vi "RT 16 bit ADC DAC.vi"() -> ()   [LabVIEW 2018]
doc: "The myRIO Custom FPGA Project template acquires button data from the onboard button and displays the button value on a Boolean indicator. The SYS.RDY indicator shows the FPGA status."
uses:
  <vilib>/FPGAPlugInAG/myRIO-1900/niLvFpga_Open_myRIO-1900.vi
  <vilib>/rvi/interface/common/dynamic/niFpgaDynamicAddResources.vi
  <vilib>/Utility/error.llb/Error Cluster From Error Code.vi
  <vilib>/rvi/errors/niLvFpgaAdjustHostInterfaceError.vi
  <vilib>/FPGAPlugInAG/Dynamic/niLvFpga_Close_Dynamic.vi
  <vilib>/rvi/interface/nirviOpenFPGA/nirviOpenFPGA.xnode
  PCB Design/16Bit_ADC_DAC/FPGA Bitfiles/ASPE2019StudentC_FPGATarget_FPGASPI_IX3lee3yG5A.lvbitx
  PCB Design/16Bit_ADC_DAC/FPGA_SPI.vi
  <vilib>/rvi/interface/nirviReadWriteControl/nirviReadWriteControl.xnode
  <vilib>/rvi/interface/nirviCloseFPGA/nirviCloseFPGA.xnode
  NiFpgaLv.dll
  <vilib>/rvi/interface/Simulation/niFpgaSimulationCallBeginRW.vi
panel:
  out "avg. loop rate (kHz)":dbl
  in  "time delay":u32=1
  out "G4":dbl(graph)
  out "G3":dbl(graph)
  out "G2":dbl(graph)
  in  "Tab Control":T1(tab)
  in  "CH1":bool[](array[boolean])=[FALSE, FALSE, FALSE, FALSE, FALSE, TRUE, FALSE, FALSE, FALSE, FALSE, FALSE, FALSE, FALSE, FALSE, FALSE, FALSE]
  in  "CH1":bool[](array[boolean])=[FALSE, FALSE, FALSE, TRUE, FALSE, TRUE, FALSE, FALSE, FALSE, FALSE, FALSE, FALSE, FALSE, FALSE, FALSE, FALSE]
  in  "CH2":bool[](array[boolean])=[FALSE, FALSE, FALSE, TRUE, FALSE, TRUE, FALSE, FALSE, FALSE, FALSE, FALSE, FALSE, FALSE, FALSE, FALSE, FALSE]
  in  "CH2":bool[](array[boolean])=[FALSE, FALSE, FALSE, TRUE, FALSE, TRUE, FALSE, FALSE, FALSE, FALSE, FALSE, FALSE, FALSE, FALSE, FALSE, FALSE]
  in  "CH3":bool[](array[boolean])=[FALSE, FALSE, TRUE, FALSE, FALSE, TRUE, FALSE, FALSE, FALSE, FALSE, FALSE, FALSE, FALSE, FALSE, FALSE, FALSE]
  in  "CH1":bool[](array[boolean])=[FALSE, FALSE, FALSE, FALSE, FALSE, TRUE, FALSE, FALSE, FALSE, FALSE, FALSE, FALSE, FALSE, FALSE, FALSE, FALSE]
  in  "CH2":bool[](array[boolean])=[FALSE, FALSE, FALSE, TRUE, FALSE, TRUE, FALSE, FALSE, FALSE, FALSE, FALSE, FALSE, FALSE, FALSE, FALSE, FALSE]
  in  "CH3":bool[](array[boolean])=[FALSE, FALSE, TRUE, FALSE, FALSE, TRUE, FALSE, FALSE, FALSE, FALSE, FALSE, FALSE, FALSE, FALSE, FALSE, FALSE]
  in  "CH4":bool[](array[boolean])=[FALSE, FALSE, TRUE, TRUE, FALSE, TRUE, FALSE, FALSE, FALSE, FALSE, FALSE, FALSE, FALSE, FALSE, FALSE, FALSE]
  in  "CH1":bool[](array[boolean])=[FALSE, FALSE, FALSE, FALSE, FALSE, TRUE, FALSE, FALSE, FALSE, FALSE, FALSE, FALSE, FALSE, FALSE, FALSE, FALSE]
  out "G1":dbl(graph)=0.00030517112470818
  in  "Amplitude":dbl=1.0 format="%0.3p"
  in  "samples per cycle":u32=1000
  out "Freq (kHz)":dbl=0.0007431959564541213 format="%.7g"
  in  "stop":bool
  # "ADC settings:"
  # "DAC settings:"
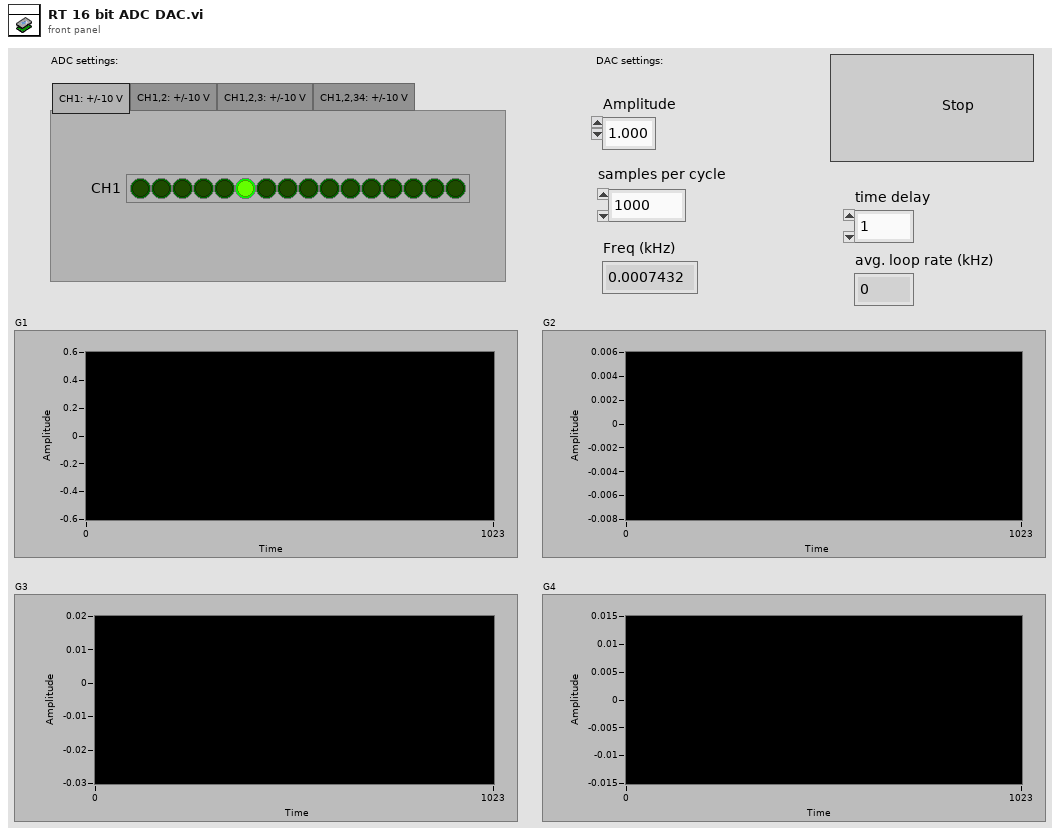
[diagram p1: front panel]
types:
  T1 = enum32{"CH1: +/-10 V", "CH1,2: +/-10 V", "CH1,2,3: +/-10 V", "CH1,2,34: +/-10 V"}
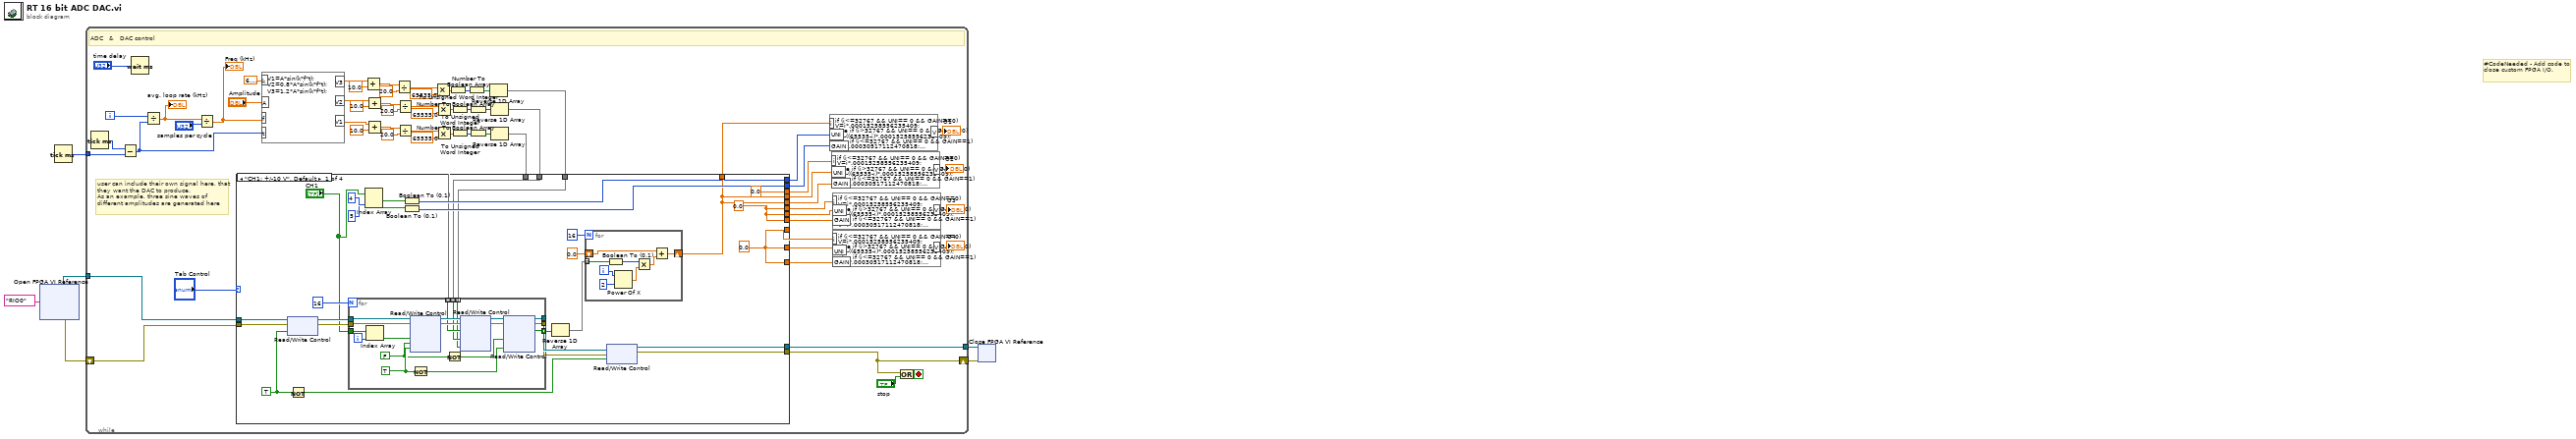
[diagram p0: block diagram]
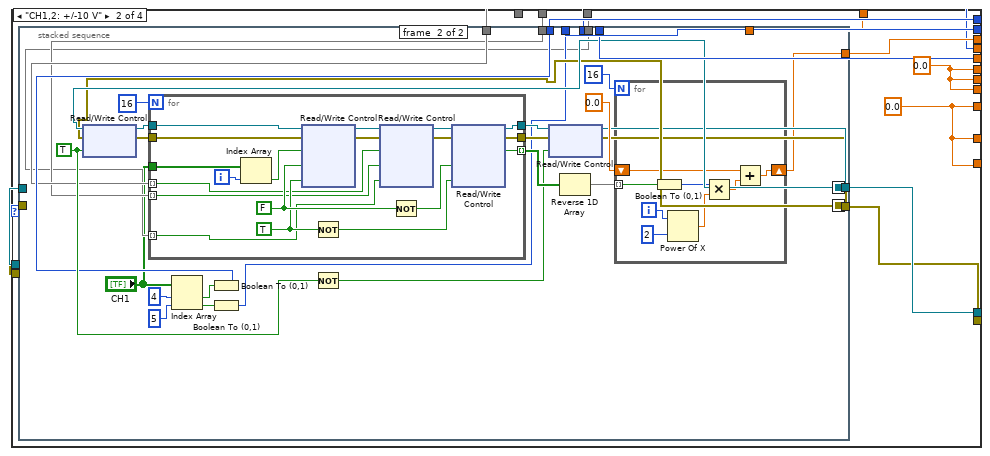
[diagram p2: hidden frame]
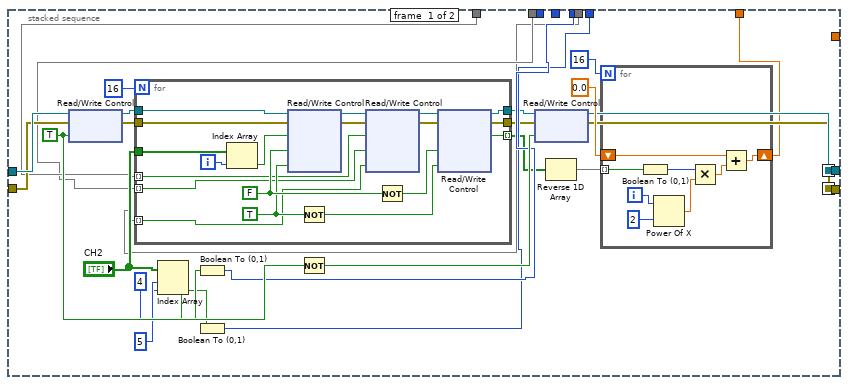
[diagram p3: hidden frame]
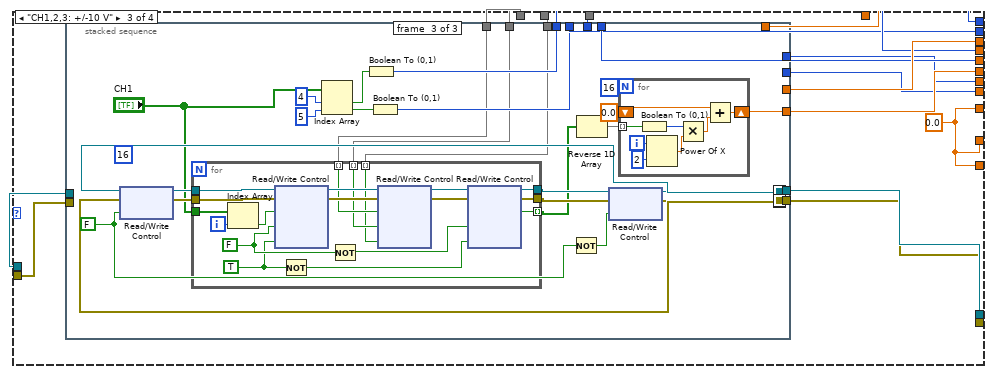
[diagram p4: hidden frame]
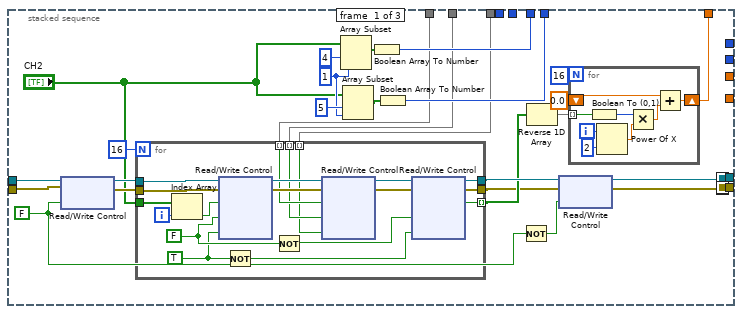
[diagram p5: hidden frame]
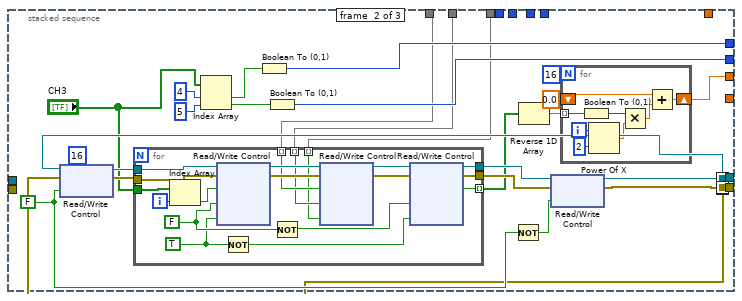
[diagram p6: hidden frame]
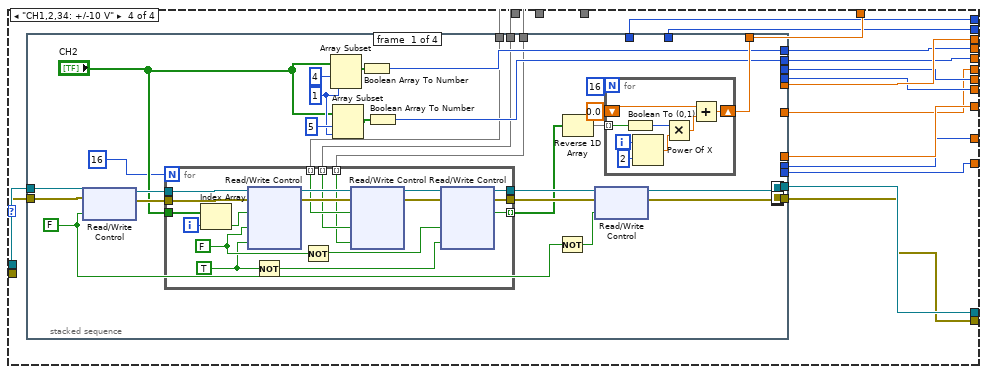
[diagram p7: hidden frame]
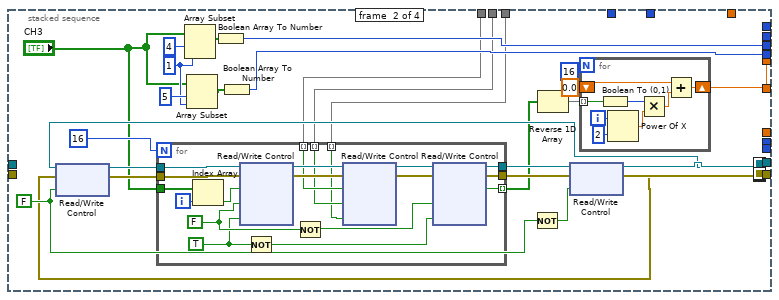
[diagram p8: hidden frame]
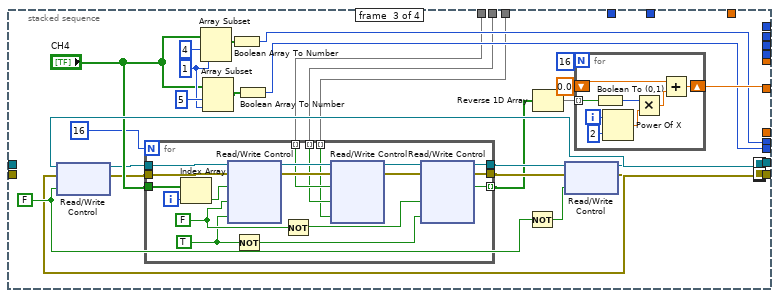
[diagram p9: hidden frame]
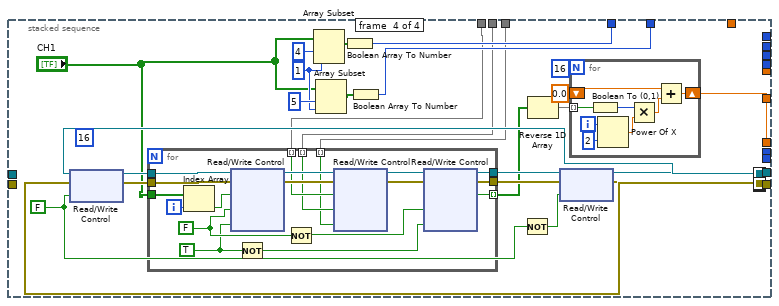
[diagram p10: hidden frame]
diagram:
  # "#CodeNeeded - Add code to close custom FPGA I/O."
  n1 = xnode "Open FPGA VI Reference"("resource name"=tag "RIO0") -> ("FPGA VI Reference Out"=w5:refnum<k20>, "error out"=w4:errorcluster)  [unwired: 1 in]
  n2 = Tick Count (ms)() -> (millisecond timer value=w2:u32)
  n3 = while {
    shift-right: [w56] -> w6
    shift-left: w4 -> [w61]
    tunnel: w2 -> [w67]
    tunnel: w5 -> [w62]
    tunnel: [w57] -> w1
    i -> [w63]
    stop <- w68 stop-if-true
    # "user can include their own signal here, that \nthey want the DAC to produce.\nAs an example, three sine waves of \ndifferent amplitudes are generated here"
    # "ADC   &   DAC control"
    n4 = Tick Count (ms)() -> (millisecond timer value=w65:u32)
    n5 = Subtract(x=w65, y=w67) -> (x-y=w53:u32)
    n6 = Wait (ms)(milliseconds to wait="time delay") -> ()  [unwired: 1 out]
    n7 = Divide(x=w63, y=w53) -> (x/y=w64:dbl)
    "avg. loop rate (kHz)" <- w64
    n8 = Divide(x=w64, y="samples per cycle") -> (x/y=w58:dbl)
    "Freq (kHz)" <- w58
    n9 = formula code="V1=A*sin(k*f*t);\nV2=0.8*A*sin(k*f*t);\nV3=1.2*A*sin(k*f*t);"("t"=w53, "f"=w58, "A"="Amplitude", "k"=6.283185307179586 ("input variable")) -> ("V1"=w25:dbl, "V3"=w44:dbl, "V2"=w34:dbl)
    n10 = Add(x=w44, y=10.0) -> (x+y=w50:dbl)
    n11 = Add(x=w34, y=10.0) -> (x+y=w40:dbl)
    n12 = Add(x=w25, y=10.0) -> (x+y=w31:dbl)
    n13 = Divide(x=w50, y=20.0) -> (x/y=w46:dbl)
    n14 = Divide(x=w40, y=20.0) -> (x/y=w36:dbl)
    n15 = Divide(x=w31, y=20.0) -> (x/y=w27:dbl)
    n16 = Multiply(x=w46, y=65535.0) -> (x*y=w47:dbl)
    n17 = Multiply(x=w36, y=65535.0) -> (x*y=w37:dbl)
    n18 = Multiply(x=w27, y=65535.0) -> (x*y=w28:dbl)
    n19 = To Unsigned Word Integer(number=w47) -> (unsigned 16bit integer=w48:u16)
    n20 = To Unsigned Word Integer(number=w37) -> (unsigned 16bit integer=w38:u16)
    n21 = To Unsigned Word Integer(number=w28) -> (unsigned 16bit integer=w29:u16)
    n22 = Number To Boolean Array(number=w48) -> (Boolean array=w45:bool[])
    n23 = Number To Boolean Array(number=w38) -> (Boolean array=w35:bool[])
    n24 = Number To Boolean Array(number=w29) -> (Boolean array=w26:bool[])
    n25 = Reverse 1D Array(array=w45) -> (reversed array=w43:bool[])
    n26 = Reverse 1D Array(array=w35) -> (reversed array=w24:bool[])
    n27 = Reverse 1D Array(array=w26) -> (reversed array=w23:bool[])
    n28 = case shown="\"CH1: +/-10 V\", Default" "Tab Control" {
      tunnel: w62 -> [w88 w140 w263 w440]
      tunnel: w61 -> [w87 w139 w262 w439]
      tunnel: [w84 w134 w259 w438] -> w22
      tunnel: [w90 w138 w261 w435] -> w57
      tunnel: [w89 w137 w260 w434] -> w56
      tunnel: [0.0 w133 w258 w437] -> w12
      tunnel: [w83 w130 w257 w425] -> w17
      tunnel: [w82 w129 w250 w436] -> w21
      tunnel: [w77 w136 w252 w427] -> w9
      tunnel: [w85 w135 w251 w426] -> w8
      tunnel: [w84 w132 w256 w433] -> w11
      tunnel: [w84 w131 w255 w432] -> w10
      tunnel: [w83 w130 w254 w431] -> w16
      tunnel: [w83 w130 w253 w430] -> w15
      tunnel: [w82 w129 w250 w429] -> w20
      tunnel: [w82 w129 w250 w428] -> w19
      tunnel: w23 -> [w73 w128 w249 w424]
      tunnel: w24 -> [w71 w127 w248 w423]
      tunnel: w43 -> [w70 w126 w247 w422]
      frame "CH1: +/-10 V", Default {
        w82 = 0.0
        w83 = 0.0
        w74 = TRUE ("CS")
        n29 = xnode "Read/Write Control"("FPGA VI Reference In"=w88, "error in"=w87, "CS"=w74) -> ("FPGA VI Reference Out"=w97:refnum<k20>, "error out"=w98:errorcluster)
        n30 = Not(x=w74) -> (.not. x?=w75:bool)
        n31 = for {
          N: 16 -> [_]
          tunnel: w97 -> [w125]
          tunnel: w98 -> [w124]
          tunnel: [w123] -> w96
          tunnel: [w122] -> w95
          tunnel: "CH1" -> [w119]
          tunnel: w73 -> [w112] mode=indexing
          tunnel: [w109] -> w72 mode=indexing
          tunnel: w71 -> [w108] mode=indexing
          tunnel: w70 -> [w107] mode=indexing
          i -> [w121]
          w110 = FALSE ("CLK")
          w114 = TRUE ("CLK")
          n32 = Index Array(array=w119, index=w121) -> (element=w120:bool)
          n33 = xnode "Read/Write Control"("FPGA VI Reference In"=w125, "error in"=w124, "MOSI1"=w120, "CLK2"=w110, "CLK1"=w114) -> ("FPGA VI Reference Out"=w118:refnum<k20>, "error out"=w117:errorcluster)
          n34 = Not(x=w114) -> (.not. x?=w113:bool)
          n35 = Not(x=w110) -> (.not. x?=w111:bool)
          n36 = xnode "Read/Write Control"("FPGA VI Reference In"=w118, "error in"=w117, "MOSI2"=w112, "MOSI3"=w108, "MOSI4"=w107) -> ("FPGA VI Reference Out"=w116:refnum<k20>, "error out"=w115:errorcluster)
          n37 = xnode "Read/Write Control"("FPGA VI Reference In"=w116, "error in"=w115, "CLK2"=w111, "CLK1"=w113) -> ("FPGA VI Reference Out"=w123:refnum<k20>, "error out"=w122:errorcluster, "MISO1"=w109:bool)
        }
        n38 = Index Array(array="CH1", index #1=4 ("index"), index #2=5 ("index")) -> (element #1=w78:bool, element #2=w76:bool)
        n39 = Boolean To (0,1)(Boolean=w78) -> (0, 1=w77:i16)
        n40 = Boolean To (0,1)(Boolean=w76) -> (0, 1=w85:i16)
        n41 = Reverse 1D Array(array=w72) -> (reversed array=w91:bool[])
        n42 = for {
          N: 16 -> [_]
          shift-right: [w104] -> w84
          shift-left: 0.0 -> [w105]
          tunnel: w91 -> [w99] mode=indexing
          i -> [w100]
          n43 = Boolean To (0,1)(Boolean=w99) -> (0, 1=w106:i16)
          n44 = Power Of X(1:2 ("y"), 2:w100) -> (0:w102:dbl)
          n45 = Multiply(x=w106, y=w102) -> (x*y=w103:dbl)
          n46 = Add(x=w105, y=w103) -> (x+y=w104:dbl)
        }
        n47 = xnode "Read/Write Control"("FPGA VI Reference In"=w96, "error in"=w95, "CS"=w75) -> ("FPGA VI Reference Out"=w90:refnum<k20>, "error out"=w89:errorcluster)
      }
      frame "CH1,2: +/-10 V" {
        w129 = 0.0
        w130 = 0.0
        n48 = stacked-sequence {
          seq-local: [w158 _] -> [_ w208]
          seq-local: [w157 _] -> [_ w207]
          tunnel: [w154 _] -> w134
          tunnel: [_ w199] -> w136
          tunnel: [_ w198] -> w135
          tunnel: [_ w204] -> w133
          tunnel: [_ w206] -> w138
          tunnel: [_ w205] -> w137
          tunnel: [w148 _] -> w132
          tunnel: [w147 _] -> w131
          tunnel: w140 -> [w156 _]
          tunnel: w139 -> [w155 _]
          tunnel: w128 -> [w144 w197]
          tunnel: w127 -> [w142 w196]
          tunnel: w126 -> [w141 w195]
          frame #0 {
            w159 = TRUE ("CS")
            n49 = xnode "Read/Write Control"("FPGA VI Reference In"=w156, "error in"=w155, "CS"=w159) -> ("FPGA VI Reference Out"=w165:refnum<k20>, "error out"=w166:errorcluster)
            n50 = for {
              N: 16 -> [_]
              tunnel: w165 -> [w183]
              tunnel: w166 -> [w182]
              tunnel: "CH2" -> [w179]
              tunnel: [w185] -> w146
              tunnel: [w184] -> w145
              tunnel: w144 -> [w181] mode=indexing
              tunnel: [w177] -> w143 mode=indexing
              tunnel: w142 -> [w176] mode=indexing
              tunnel: w141 -> [w175] mode=indexing
              i -> [w180]
              w193 = FALSE ("CLK")
              w192 = TRUE ("CLK")
              n51 = Index Array(array=w179, index=w180) -> (element=w178:bool)
              n52 = xnode "Read/Write Control"("FPGA VI Reference In"=w183, "error in"=w182, "MOSI1"=w178, "CLK2"=w193, "CLK1"=w192) -> ("FPGA VI Reference Out"=w191:refnum<k20>, "error out"=w190:errorcluster)
              n53 = Not(x=w192) -> (.not. x?=w186:bool)
              n54 = xnode "Read/Write Control"("FPGA VI Reference In"=w191, "error in"=w190, "MOSI2"=w181, "MOSI3"=w176, "MOSI4"=w175) -> ("FPGA VI Reference Out"=w189:refnum<k20>, "error out"=w188:errorcluster)
              n55 = Not(x=w193) -> (.not. x?=w187:bool)
              n56 = xnode "Read/Write Control"("FPGA VI Reference In"=w189, "error in"=w188, "CLK2"=w187, "CLK1"=w186) -> ("FPGA VI Reference Out"=w185:refnum<k20>, "error out"=w184:errorcluster, "MISO1"=w177:bool)
            }
            n57 = Index Array(array="CH2", index #1=4 ("index"), index #2=5 ("index")) -> (element #1=w151:bool, element #2=w150:bool)
            n58 = Boolean To (0,1)(Boolean=w151) -> (0, 1=w148:i16)
            n59 = Boolean To (0,1)(Boolean=w150) -> (0, 1=w147:i16)
            n60 = Not(x=w159) -> (.not. x?=w160:bool)
            n61 = xnode "Read/Write Control"("FPGA VI Reference In"=w146, "error in"=w145, "CS"=w160) -> ("FPGA VI Reference Out"=w158:refnum<k20>, "error out"=w157:errorcluster)
            n62 = Reverse 1D Array(array=w143) -> (reversed array=w161:bool[])
            n63 = for {
              N: 16 -> [_]
              shift-right: [w172] -> w154
              shift-left: 0.0 -> [w173]
              tunnel: w161 -> [w167] mode=indexing
              i -> [w168]
              n64 = Boolean To (0,1)(Boolean=w167) -> (0, 1=w174:i16)
              n65 = Power Of X(1:2 ("y"), 2:w168) -> (0:w170:dbl)
              n66 = Multiply(x=w174, y=w170) -> (x*y=w171:dbl)
              n67 = Add(x=w173, y=w171) -> (x+y=w172:dbl)
            }
          }
          frame #1 {
            w209 = TRUE ("CS")
            n68 = xnode "Read/Write Control"("FPGA VI Reference In"=w208, "error in"=w207, "CS"=w209) -> ("FPGA VI Reference Out"=w218:refnum<k20>, "error out"=w219:errorcluster)
            n69 = for {
              N: 16 -> [_]
              tunnel: w218 -> [w246]
              tunnel: w219 -> [w245]
              tunnel: [w244] -> w211 mode=indexing
              tunnel: [w243] -> w217
              tunnel: [w242] -> w216
              tunnel: "CH1" -> [w239]
              tunnel: w197 -> [w232] mode=indexing
              tunnel: w196 -> [w229] mode=indexing
              tunnel: w195 -> [w228] mode=indexing
              i -> [w241]
              w238 = FALSE ("CLK")
              w237 = TRUE ("CLK")
              n70 = Index Array(array=w239, index=w241) -> (element=w240:bool)
              n71 = xnode "Read/Write Control"("FPGA VI Reference In"=w246, "error in"=w245, "MOSI1"=w240, "CLK2"=w238, "CLK1"=w237) -> ("FPGA VI Reference Out"=w236:refnum<k20>, "error out"=w235:errorcluster)
              n72 = Not(x=w237) -> (.not. x?=w230:bool)
              n73 = xnode "Read/Write Control"("FPGA VI Reference In"=w236, "error in"=w235, "MOSI2"=w232, "MOSI3"=w229, "MOSI4"=w228) -> ("FPGA VI Reference Out"=w234:refnum<k20>, "error out"=w233:errorcluster)
              n74 = Not(x=w238) -> (.not. x?=w231:bool)
              n75 = xnode "Read/Write Control"("FPGA VI Reference In"=w234, "error in"=w233, "CLK2"=w231, "CLK1"=w230) -> ("FPGA VI Reference Out"=w243:refnum<k20>, "error out"=w242:errorcluster, "MISO1"=w244:bool)
            }
            n76 = Index Array(array="CH1", index #1=4 ("index"), index #2=5 ("index")) -> (element #1=w201:bool, element #2=w200:bool)
            n77 = Boolean To (0,1)(Boolean=w201) -> (0, 1=w199:i16)
            n78 = Boolean To (0,1)(Boolean=w200) -> (0, 1=w198:i16)
            n79 = Not(x=w209) -> (.not. x?=w210:bool)
            n80 = xnode "Read/Write Control"("FPGA VI Reference In"=w217, "error in"=w216, "CS"=w210) -> ("FPGA VI Reference Out"=w206:refnum<k20>, "error out"=w205:errorcluster)
            n81 = Reverse 1D Array(array=w211) -> (reversed array=w212:bool[])
            n82 = for {
              N: 16 -> [_]
              shift-right: [w225] -> w204
              shift-left: 0.0 -> [w226]
              tunnel: w212 -> [w220] mode=indexing
              i -> [w221]
              n83 = Boolean To (0,1)(Boolean=w220) -> (0, 1=w227:i16)
              n84 = Power Of X(1:2 ("y"), 2:w221) -> (0:w223:dbl)
              n85 = Multiply(x=w227, y=w223) -> (x*y=w224:dbl)
              n86 = Add(x=w226, y=w224) -> (x+y=w225:dbl)
            }
          }
        }
      }
      frame "CH1,2,3: +/-10 V" {
        w250 = 0.0
        n87 = stacked-sequence {
          seq-local: [w285 _ _] -> [_ w335 _]
          seq-local: [w284 _ _] -> [_ w334 _]
          seq-local: [_ w337 _] -> [_ _ w389]
          seq-local: [_ w336 _] -> [_ _ w388]
          tunnel: [w283 _ _] -> w259
          tunnel: [_ w333 _] -> w258
          tunnel: [_ _ w387] -> w261
          tunnel: [_ _ w386] -> w260
          tunnel: [_ _ w385] -> w257
          tunnel: w263 -> [w282 _ _]
          tunnel: w262 -> [w281 _ _]
          tunnel: [w275 _ _] -> w256
          tunnel: [w274 _ _] -> w255
          tunnel: [_ w328 _] -> w254
          tunnel: [_ w327 _] -> w253
          tunnel: [_ _ w384] -> w252
          tunnel: [_ _ w383] -> w251
          tunnel: w249 -> [w270 w320 w375]
          tunnel: w248 -> [w265 w319 w371]
          tunnel: w247 -> [w264 w318 w370]
          frame #0 {
            w276 = 1 ("length")
            w286 = FALSE ("CS")
            n88 = xnode "Read/Write Control"("FPGA VI Reference In"=w282, "error in"=w281, "CS"=w286) -> ("FPGA VI Reference Out"=w273:refnum<k20>, "error out"=w272:errorcluster)
            n89 = for {
              N: 16 -> [_]
              tunnel: w273 -> [w309]
              tunnel: w272 -> [w308]
              tunnel: [w307] -> w268 mode=indexing
              tunnel: [w306] -> w269
              tunnel: [w305] -> w267
              tunnel: "CH2" -> [w302]
              tunnel: w270 -> [w295] mode=indexing
              tunnel: w265 -> [w292] mode=indexing
              tunnel: w264 -> [w291] mode=indexing
              i -> [w304]
              w301 = FALSE ("CLK")
              w300 = TRUE ("CLK")
              n90 = Index Array(array=w302, index=w304) -> (element=w303:bool)
              n91 = xnode "Read/Write Control"("FPGA VI Reference In"=w309, "error in"=w308, "MOSI1"=w303, "CLK2"=w301, "CLK1"=w300) -> ("FPGA VI Reference Out"=w299:refnum<k20>, "error out"=w298:errorcluster)
              n92 = Not(x=w300) -> (.not. x?=w293:bool)
              n93 = Not(x=w301) -> (.not. x?=w294:bool)
              n94 = xnode "Read/Write Control"("FPGA VI Reference In"=w299, "error in"=w298, "MOSI2"=w295, "MOSI3"=w292, "MOSI4"=w291) -> ("FPGA VI Reference Out"=w297:refnum<k20>, "error out"=w296:errorcluster)
              n95 = xnode "Read/Write Control"("FPGA VI Reference In"=w297, "error in"=w296, "CLK2"=w294, "CLK1"=w293) -> ("FPGA VI Reference Out"=w306:refnum<k20>, "error out"=w305:errorcluster, "MISO1"=w307:bool)
            }
            n96 = Array Subset(array="CH2", index=4, length=w276) -> (w278:bool[])
            n97 = Array Subset(array="CH2", index=5, length=w276) -> (w277:bool[])
            n98 = Boolean Array To Number(Boolean array=w278) -> (number=w275:u32)
            n99 = Boolean Array To Number(Boolean array=w277) -> (number=w274:u32)
            n100 = Not(x=w286) -> (.not. x?=w287:bool)
            n101 = Reverse 1D Array(array=w268) -> (reversed array=w288:bool[])
            n102 = xnode "Read/Write Control"("FPGA VI Reference In"=w269, "error in"=w267, "CS"=w287) -> ("FPGA VI Reference Out"=w285:refnum<k20>, "error out"=w284:errorcluster)
            n103 = for {
              N: 16 -> [_]
              shift-right: [w310] -> w283
              shift-left: 0.0 -> [w316]
              tunnel: w288 -> [w311] mode=indexing
              i -> [w312]
              n104 = Boolean To (0,1)(Boolean=w311) -> (0, 1=w317:i16)
              n105 = Power Of X(1:2 ("y"), 2:w312) -> (0:w314:dbl)
              n106 = Multiply(x=w317, y=w314) -> (x*y=w315:dbl)
              n107 = Add(x=w316, y=w315) -> (x+y=w310:dbl)
            }
          }
          frame #1 {
            w338 = FALSE ("CS")
            (unwired) 16
            n108 = xnode "Read/Write Control"("FPGA VI Reference In"=w335, "error in"=w334, "CS"=w338) -> ("FPGA VI Reference Out"=w326:refnum<k20>, "error out"=w325:errorcluster)
            n109 = for {
              tunnel: w326 -> [w361]
              tunnel: w325 -> [w360]
              tunnel: [w359] -> w321 mode=indexing
              tunnel: [w358] -> w323
              tunnel: [w357] -> w322
              tunnel: "CH3" -> [w354]
              tunnel: w320 -> [w347] mode=indexing
              tunnel: w319 -> [w344] mode=indexing
              tunnel: w318 -> [w343] mode=indexing
              i -> [w356]
              w353 = FALSE ("CLK")
              w352 = TRUE ("CLK")
              n110 = Index Array(array=w354, index=w356) -> (element=w355:bool)
              n111 = xnode "Read/Write Control"("FPGA VI Reference In"=w361, "error in"=w360, "MOSI1"=w355, "CLK2"=w353, "CLK1"=w352) -> ("FPGA VI Reference Out"=w351:refnum<k20>, "error out"=w350:errorcluster)
              n112 = Not(x=w352) -> (.not. x?=w345:bool)
              n113 = Not(x=w353) -> (.not. x?=w346:bool)
              n114 = xnode "Read/Write Control"("FPGA VI Reference In"=w351, "error in"=w350, "MOSI2"=w347, "MOSI3"=w344, "MOSI4"=w343) -> ("FPGA VI Reference Out"=w349:refnum<k20>, "error out"=w348:errorcluster)
              n115 = xnode "Read/Write Control"("FPGA VI Reference In"=w349, "error in"=w348, "CLK2"=w346, "CLK1"=w345) -> ("FPGA VI Reference Out"=w358:refnum<k20>, "error out"=w357:errorcluster, "MISO1"=w359:bool)
            }
            n116 = Index Array(array="CH3", index #1=4 ("index"), index #2=5 ("index")) -> (element #1=w330:bool, element #2=w329:bool)
            n117 = Boolean To (0,1)(Boolean=w330) -> (0, 1=w328:i16)
            n118 = Boolean To (0,1)(Boolean=w329) -> (0, 1=w327:i16)
            n119 = Not(x=w338) -> (.not. x?=w339:bool)
            n120 = Reverse 1D Array(array=w321) -> (reversed array=w340:bool[])
            n121 = xnode "Read/Write Control"("FPGA VI Reference In"=w323, "error in"=w322, "CS"=w339) -> ("FPGA VI Reference Out"=w337:refnum<k20>, "error out"=w336:errorcluster)
            n122 = for {
              N: 16 -> [_]
              shift-right: [w367] -> w333
              shift-left: 0.0 -> [w368]
              tunnel: w340 -> [w362] mode=indexing
              i -> [w363]
              n123 = Boolean To (0,1)(Boolean=w362) -> (0, 1=w369:i16)
              n124 = Power Of X(1:2 ("y"), 2:w363) -> (0:w365:dbl)
              n125 = Multiply(x=w369, y=w365) -> (x*y=w366:dbl)
              n126 = Add(x=w368, y=w366) -> (x+y=w367:dbl)
            }
          }
          frame #2 {
            w390 = FALSE ("CS")
            (unwired) 16
            n127 = xnode "Read/Write Control"("FPGA VI Reference In"=w389, "error in"=w388, "CS"=w390) -> ("FPGA VI Reference Out"=w374:refnum<k20>, "error out"=w373:errorcluster)
            n128 = for {
              tunnel: w374 -> [w413]
              tunnel: w373 -> [w412]
              tunnel: [w411] -> w376 mode=indexing
              tunnel: [w410] -> w378
              tunnel: [w409] -> w377
              tunnel: "CH1" -> [w406]
              tunnel: w375 -> [w399] mode=indexing
              tunnel: w371 -> [w396] mode=indexing
              tunnel: w370 -> [w395] mode=indexing
              i -> [w408]
              w405 = FALSE ("CLK")
              w404 = TRUE ("CLK")
              n129 = Index Array(array=w406, index=w408) -> (element=w407:bool)
              n130 = xnode "Read/Write Control"("FPGA VI Reference In"=w413, "error in"=w412, "MOSI1"=w407, "CLK2"=w405, "CLK1"=w404) -> ("FPGA VI Reference Out"=w403:refnum<k20>, "error out"=w402:errorcluster)
              n131 = Not(x=w404) -> (.not. x?=w397:bool)
              n132 = Not(x=w405) -> (.not. x?=w398:bool)
              n133 = xnode "Read/Write Control"("FPGA VI Reference In"=w403, "error in"=w402, "MOSI2"=w399, "MOSI3"=w396, "MOSI4"=w395) -> ("FPGA VI Reference Out"=w401:refnum<k20>, "error out"=w400:errorcluster)
              n134 = xnode "Read/Write Control"("FPGA VI Reference In"=w401, "error in"=w400, "CLK2"=w398, "CLK1"=w397) -> ("FPGA VI Reference Out"=w410:refnum<k20>, "error out"=w409:errorcluster, "MISO1"=w411:bool)
            }
            n135 = Index Array(array="CH1", index #1=4 ("index"), index #2=5 ("index")) -> (element #1=w380:bool, element #2=w379:bool)
            n136 = Boolean To (0,1)(Boolean=w380) -> (0, 1=w384:i16)
            n137 = Boolean To (0,1)(Boolean=w379) -> (0, 1=w383:i16)
            n138 = Not(x=w390) -> (.not. x?=w391:bool)
            n139 = Reverse 1D Array(array=w376) -> (reversed array=w392:bool[])
            n140 = xnode "Read/Write Control"("FPGA VI Reference In"=w378, "error in"=w377, "CS"=w391) -> ("FPGA VI Reference Out"=w387:refnum<k20>, "error out"=w386:errorcluster)
            n141 = for {
              N: 16 -> [_]
              shift-right: [w419] -> w385
              shift-left: 0.0 -> [w420]
              tunnel: w392 -> [w414] mode=indexing
              i -> [w415]
              n142 = Boolean To (0,1)(Boolean=w414) -> (0, 1=w421:i16)
              n143 = Power Of X(1:2 ("y"), 2:w415) -> (0:w417:dbl)
              n144 = Multiply(x=w421, y=w417) -> (x*y=w418:dbl)
              n145 = Add(x=w420, y=w418) -> (x+y=w419:dbl)
            }
          }
        }
      }
      frame "CH1,2,34: +/-10 V" {
        n146 = stacked-sequence {
          seq-local: [w462 _ _ _] -> [_ w514 _ _]
          seq-local: [w461 _ _ _] -> [_ w513 _ _]
          seq-local: [_ w516 _ _] -> [_ _ w570 _]
          seq-local: [_ w515 _ _] -> [_ _ w569 _]
          seq-local: [_ _ w568 _] -> [_ _ _ w623]
          seq-local: [_ _ w567 _] -> [_ _ _ w622]
          tunnel: [w460 _ _ _] -> w438
          tunnel: [_ w512 _ _] -> w437
          tunnel: [_ _ w566 _] -> w425
          tunnel: [_ _ _ w621] -> w435
          tunnel: [_ _ _ w620] -> w434
          tunnel: [_ _ _ w619] -> w436
          tunnel: w440 -> [w459 _ _ _]
          tunnel: w439 -> [w458 _ _ _]
          tunnel: [w452 _ _ _] -> w433
          tunnel: [w451 _ _ _] -> w432
          tunnel: [_ w506 _ _] -> w431
          tunnel: [_ w505 _ _] -> w430
          tunnel: [_ _ w560 _] -> w429
          tunnel: [_ _ w559 _] -> w428
          tunnel: [_ _ _ w613] -> w427
          tunnel: [_ _ _ w612] -> w426
          tunnel: w424 -> [w446 w500 w554 w608]
          tunnel: w423 -> [w442 w496 w550 w604]
          tunnel: w422 -> [w441 w495 w549 w603]
          frame #0 {
            w453 = 1 ("length")
            w463 = FALSE ("CS")
            n147 = xnode "Read/Write Control"("FPGA VI Reference In"=w459, "error in"=w458, "CS"=w463) -> ("FPGA VI Reference Out"=w450:refnum<k20>, "error out"=w449:errorcluster)
            n148 = for {
              N: 16 -> [_]
              tunnel: w450 -> [w486]
              tunnel: w449 -> [w485]
              tunnel: [w484] -> w443 mode=indexing
              tunnel: [w483] -> w445
              tunnel: [w482] -> w444
              tunnel: "CH2" -> [w479]
              tunnel: w446 -> [w472] mode=indexing
              tunnel: w442 -> [w469] mode=indexing
              tunnel: w441 -> [w468] mode=indexing
              i -> [w481]
              w478 = FALSE ("CLK")
              w477 = TRUE ("CLK")
              n149 = Index Array(array=w479, index=w481) -> (element=w480:bool)
              n150 = xnode "Read/Write Control"("FPGA VI Reference In"=w486, "error in"=w485, "MOSI1"=w480, "CLK2"=w478, "CLK1"=w477) -> ("FPGA VI Reference Out"=w476:refnum<k20>, "error out"=w475:errorcluster)
              n151 = Not(x=w477) -> (.not. x?=w470:bool)
              n152 = Not(x=w478) -> (.not. x?=w471:bool)
              n153 = xnode "Read/Write Control"("FPGA VI Reference In"=w476, "error in"=w475, "MOSI2"=w472, "MOSI3"=w469, "MOSI4"=w468) -> ("FPGA VI Reference Out"=w474:refnum<k20>, "error out"=w473:errorcluster)
              n154 = xnode "Read/Write Control"("FPGA VI Reference In"=w474, "error in"=w473, "CLK2"=w471, "CLK1"=w470) -> ("FPGA VI Reference Out"=w483:refnum<k20>, "error out"=w482:errorcluster, "MISO1"=w484:bool)
            }
            n155 = Array Subset(array="CH2", index=4, length=w453) -> (w455:bool[])
            n156 = Array Subset(array="CH2", index=5, length=w453) -> (w454:bool[])
            n157 = Boolean Array To Number(Boolean array=w455) -> (number=w452:u32)
            n158 = Boolean Array To Number(Boolean array=w454) -> (number=w451:u32)
            n159 = Not(x=w463) -> (.not. x?=w464:bool)
            n160 = Reverse 1D Array(array=w443) -> (reversed array=w465:bool[])
            n161 = xnode "Read/Write Control"("FPGA VI Reference In"=w445, "error in"=w444, "CS"=w464) -> ("FPGA VI Reference Out"=w462:refnum<k20>, "error out"=w461:errorcluster)
            n162 = for {
              N: 16 -> [_]
              shift-right: [w492] -> w460
              shift-left: 0.0 -> [w493]
              tunnel: w465 -> [w487] mode=indexing
              i -> [w488]
              n163 = Boolean To (0,1)(Boolean=w487) -> (0, 1=w494:i16)
              n164 = Power Of X(1:2 ("y"), 2:w488) -> (0:w490:dbl)
              n165 = Multiply(x=w494, y=w490) -> (x*y=w491:dbl)
              n166 = Add(x=w493, y=w491) -> (x+y=w492:dbl)
            }
          }
          frame #1 {
            w507 = 1 ("length")
            w517 = FALSE ("CS")
            n167 = xnode "Read/Write Control"("FPGA VI Reference In"=w514, "error in"=w513, "CS"=w517) -> ("FPGA VI Reference Out"=w499:refnum<k20>, "error out"=w498:errorcluster)
            n168 = for {
              N: 16 -> [_]
              tunnel: w499 -> [w540]
              tunnel: w498 -> [w539]
              tunnel: [w538] -> w501 mode=indexing
              tunnel: [w537] -> w503
              tunnel: [w536] -> w502
              tunnel: "CH3" -> [w533]
              tunnel: w500 -> [w526] mode=indexing
              tunnel: w496 -> [w523] mode=indexing
              tunnel: w495 -> [w522] mode=indexing
              i -> [w535]
              w532 = FALSE ("CLK")
              w531 = TRUE ("CLK")
              n169 = Index Array(array=w533, index=w535) -> (element=w534:bool)
              n170 = xnode "Read/Write Control"("FPGA VI Reference In"=w540, "error in"=w539, "MOSI1"=w534, "CLK2"=w532, "CLK1"=w531) -> ("FPGA VI Reference Out"=w530:refnum<k20>, "error out"=w529:errorcluster)
              n171 = Not(x=w531) -> (.not. x?=w524:bool)
              n172 = Not(x=w532) -> (.not. x?=w525:bool)
              n173 = xnode "Read/Write Control"("FPGA VI Reference In"=w530, "error in"=w529, "MOSI2"=w526, "MOSI3"=w523, "MOSI4"=w522) -> ("FPGA VI Reference Out"=w528:refnum<k20>, "error out"=w527:errorcluster)
              n174 = xnode "Read/Write Control"("FPGA VI Reference In"=w528, "error in"=w527, "CLK2"=w525, "CLK1"=w524) -> ("FPGA VI Reference Out"=w537:refnum<k20>, "error out"=w536:errorcluster, "MISO1"=w538:bool)
            }
            n175 = Array Subset(array="CH3", index=4, length=w507) -> (w509:bool[])
            n176 = Array Subset(array="CH3", index=5, length=w507) -> (w508:bool[])
            n177 = Boolean Array To Number(Boolean array=w509) -> (number=w506:u32)
            n178 = Boolean Array To Number(Boolean array=w508) -> (number=w505:u32)
            n179 = Not(x=w517) -> (.not. x?=w518:bool)
            n180 = Reverse 1D Array(array=w501) -> (reversed array=w519:bool[])
            n181 = xnode "Read/Write Control"("FPGA VI Reference In"=w503, "error in"=w502, "CS"=w518) -> ("FPGA VI Reference Out"=w516:refnum<k20>, "error out"=w515:errorcluster)
            n182 = for {
              N: 16 -> [_]
              shift-right: [w546] -> w512
              shift-left: 0.0 -> [w547]
              tunnel: w519 -> [w541] mode=indexing
              i -> [w542]
              n183 = Boolean To (0,1)(Boolean=w541) -> (0, 1=w548:i16)
              n184 = Power Of X(1:2 ("y"), 2:w542) -> (0:w544:dbl)
              n185 = Multiply(x=w548, y=w544) -> (x*y=w545:dbl)
              n186 = Add(x=w547, y=w545) -> (x+y=w546:dbl)
            }
          }
          frame #2 {
            w561 = 1 ("length")
            w571 = FALSE ("CS")
            n187 = xnode "Read/Write Control"("FPGA VI Reference In"=w570, "error in"=w569, "CS"=w571) -> ("FPGA VI Reference Out"=w556:refnum<k20>, "error out"=w557:errorcluster)
            n188 = for {
              N: 16 -> [_]
              tunnel: w556 -> [w594]
              tunnel: w557 -> [w593]
              tunnel: [w592] -> w551 mode=indexing
              tunnel: [w591] -> w553
              tunnel: [w590] -> w552
              tunnel: "CH4" -> [w587]
              tunnel: w554 -> [w580] mode=indexing
              tunnel: w550 -> [w577] mode=indexing
              tunnel: w549 -> [w576] mode=indexing
              i -> [w589]
              w586 = FALSE ("CLK")
              w585 = TRUE ("CLK")
              n189 = Index Array(array=w587, index=w589) -> (element=w588:bool)
              n190 = xnode "Read/Write Control"("FPGA VI Reference In"=w594, "error in"=w593, "MOSI1"=w588, "CLK2"=w586, "CLK1"=w585) -> ("FPGA VI Reference Out"=w584:refnum<k20>, "error out"=w583:errorcluster)
              n191 = Not(x=w585) -> (.not. x?=w578:bool)
              n192 = Not(x=w586) -> (.not. x?=w579:bool)
              n193 = xnode "Read/Write Control"("FPGA VI Reference In"=w584, "error in"=w583, "MOSI2"=w580, "MOSI3"=w577, "MOSI4"=w576) -> ("FPGA VI Reference Out"=w582:refnum<k20>, "error out"=w581:errorcluster)
              n194 = xnode "Read/Write Control"("FPGA VI Reference In"=w582, "error in"=w581, "CLK2"=w579, "CLK1"=w578) -> ("FPGA VI Reference Out"=w591:refnum<k20>, "error out"=w590:errorcluster, "MISO1"=w592:bool)
            }
            n195 = Array Subset(array="CH4", index=4, length=w561) -> (w563:bool[])
            n196 = Array Subset(array="CH4", index=5, length=w561) -> (w562:bool[])
            n197 = Boolean Array To Number(Boolean array=w563) -> (number=w560:u32)
            n198 = Boolean Array To Number(Boolean array=w562) -> (number=w559:u32)
            n199 = Not(x=w571) -> (.not. x?=w572:bool)
            n200 = Reverse 1D Array(array=w551) -> (reversed array=w573:bool[])
            n201 = xnode "Read/Write Control"("FPGA VI Reference In"=w553, "error in"=w552, "CS"=w572) -> ("FPGA VI Reference Out"=w568:refnum<k20>, "error out"=w567:errorcluster)
            n202 = for {
              N: 16 -> [_]
              shift-right: [w600] -> w566
              shift-left: 0.0 -> [w601]
              tunnel: w573 -> [w595] mode=indexing
              i -> [w596]
              n203 = Boolean To (0,1)(Boolean=w595) -> (0, 1=w602:i16)
              n204 = Power Of X(1:2 ("y"), 2:w596) -> (0:w598:dbl)
              n205 = Multiply(x=w602, y=w598) -> (x*y=w599:dbl)
              n206 = Add(x=w601, y=w599) -> (x+y=w600:dbl)
            }
          }
          frame #3 {
            w614 = 1 ("length")
            w624 = FALSE ("CS")
            (unwired) 16
            n207 = xnode "Read/Write Control"("FPGA VI Reference In"=w623, "error in"=w622, "CS"=w624) -> ("FPGA VI Reference Out"=w611:refnum<k20>, "error out"=w610:errorcluster)
            n208 = for {
              tunnel: w611 -> [w647]
              tunnel: w610 -> [w646]
              tunnel: [w645] -> w605 mode=indexing
              tunnel: [w644] -> w607
              tunnel: [w643] -> w606
              tunnel: "CH1" -> [w640]
              tunnel: w608 -> [w633] mode=indexing
              tunnel: w604 -> [w630] mode=indexing
              tunnel: w603 -> [w629] mode=indexing
              i -> [w642]
              w639 = FALSE ("CLK")
              w638 = TRUE ("CLK")
              n209 = Index Array(array=w640, index=w642) -> (element=w641:bool)
              n210 = xnode "Read/Write Control"("FPGA VI Reference In"=w647, "error in"=w646, "MOSI1"=w641, "CLK2"=w639, "CLK1"=w638) -> ("FPGA VI Reference Out"=w637:refnum<k20>, "error out"=w636:errorcluster)
              n211 = Not(x=w638) -> (.not. x?=w631:bool)
              n212 = Not(x=w639) -> (.not. x?=w632:bool)
              n213 = xnode "Read/Write Control"("FPGA VI Reference In"=w637, "error in"=w636, "MOSI2"=w633, "MOSI3"=w630, "MOSI4"=w629) -> ("FPGA VI Reference Out"=w635:refnum<k20>, "error out"=w634:errorcluster)
              n214 = xnode "Read/Write Control"("FPGA VI Reference In"=w635, "error in"=w634, "CLK2"=w632, "CLK1"=w631) -> ("FPGA VI Reference Out"=w644:refnum<k20>, "error out"=w643:errorcluster, "MISO1"=w645:bool)
            }
            n215 = Array Subset(array="CH1", index=4, length=w614) -> (w616:bool[])
            n216 = Array Subset(array="CH1", index=5, length=w614) -> (w615:bool[])
            n217 = Boolean Array To Number(Boolean array=w616) -> (number=w613:u32)
            n218 = Boolean Array To Number(Boolean array=w615) -> (number=w612:u32)
            n219 = Not(x=w624) -> (.not. x?=w625:bool)
            n220 = Reverse 1D Array(array=w605) -> (reversed array=w626:bool[])
            n221 = xnode "Read/Write Control"("FPGA VI Reference In"=w607, "error in"=w606, "CS"=w625) -> ("FPGA VI Reference Out"=w621:refnum<k20>, "error out"=w620:errorcluster)
            n222 = for {
              N: 16 -> [_]
              shift-right: [w653] -> w619
              shift-left: 0.0 -> [w654]
              tunnel: w626 -> [w648] mode=indexing
              i -> [w649]
              n223 = Boolean To (0,1)(Boolean=w648) -> (0, 1=w655:i16)
              n224 = Power Of X(1:2 ("y"), 2:w649) -> (0:w651:dbl)
              n225 = Multiply(x=w655, y=w651) -> (x*y=w652:dbl)
              n226 = Add(x=w654, y=w652) -> (x+y=w653:dbl)
            }
          }
        }
      }
    }
    n227 = formula code="if (i<=32767 && UNI== 0 && GAIN==0)\nV=i*.00015258556235409;\nelse if (i>32767 && UNI== 0 && GAIN==0)\nV=-((65535-i)*.00015258556235409);\nelse if (i<=32767 && UNI== 0 && GAIN==1)\nV=i*.00030517112470818;\nelse if (i>32767 && UNI== 0 && GAIN==1)\nV=-((65535-i)*.00030517112470818);\nelse if (i<=65535 && UNI== 1 && GAIN==0)\nV=i*.000076292781177045028;\nelse\nV=i*.00015258556235409;"("i"=w22, "GAIN"=w8, "UNI"=w9) -> ("V"=→"G1":dbl)
    n228 = formula code="if (i<=32767 && UNI== 0 && GAIN==0)\nV=i*.00015258556235409;\nelse if (i>32767 && UNI== 0 && GAIN==0)\nV=-((65535-i)*.00015258556235409);\nelse if (i<=32767 && UNI== 0 && GAIN==1)\nV=i*.00030517112470818;\nelse if (i>32767 && UNI== 0 && GAIN==1)\nV=-((65535-i)*.00030517112470818);\nelse if (i<=65535 && UNI== 1 && GAIN==0)\nV=i*.000076292781177045028;\nelse\nV=i*.00015258556235409;"("i"=w12, "GAIN"=w10, "UNI"=w11) -> ("V"=→"G2":dbl)
    n229 = formula code="if (i<=32767 && UNI== 0 && GAIN==0)\nV=i*.00015258556235409;\nelse if (i>32767 && UNI== 0 && GAIN==0)\nV=-((65535-i)*.00015258556235409);\nelse if (i<=32767 && UNI== 0 && GAIN==1)\nV=i*.00030517112470818;\nelse if (i>32767 && UNI== 0 && GAIN==1)\nV=-((65535-i)*.00030517112470818);\nelse if (i<=65535 && UNI== 1 && GAIN==0)\nV=i*.000076292781177045028;\nelse\nV=i*.00015258556235409;"("i"=w17, "GAIN"=w15, "UNI"=w16) -> ("V"=→"G3":dbl)
    n230 = formula code="if (i<=32767 && UNI== 0 && GAIN==0)\nV=i*.00015258556235409;\nelse if (i>32767 && UNI== 0 && GAIN==0)\nV=-((65535-i)*.00015258556235409);\nelse if (i<=32767 && UNI== 0 && GAIN==1)\nV=i*.00030517112470818;\nelse if (i>32767 && UNI== 0 && GAIN==1)\nV=-((65535-i)*.00030517112470818);\nelse if (i<=65535 && UNI== 1 && GAIN==0)\nV=i*.000076292781177045028;\nelse\nV=i*.00015258556235409;"("i"=w21, "GAIN"=w19, "UNI"=w20) -> ("V"=→"G4":dbl)
    n231 = Or(x=w56, y="stop") -> (x .or. y?=w68:bool)
  }
  n232 = xnode "Close FPGA VI Reference"("FPGA VI Reference In"=w1, "error in"=w6) -> ()  [unwired: 1 out]
